vi "Describe Comparison.vi"(6 "Delta":variant, 9 "Actual":variant, 10 "Expected":variant) -> (2 "Description":string)   [LabVIEW 2020]
uses:
  <vilib>/Utility/Data Type/NI_Data Type.lvlib
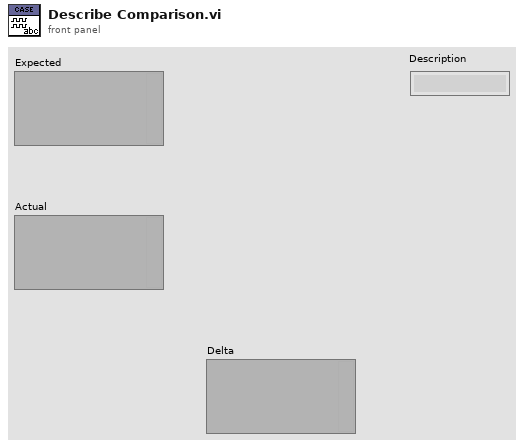
[diagram p1: front panel]
types:
  T1 = typedef "NI_Data Type.lvlib/Data Type.ctl" = enum8{"Invalid Type", "Void", "I8", "I16", "I32", "I64", "U8", "U16", "U32", "U64", "Single Float", "Double Float", "Extended Float", "Single Complex", "Double Complex", "Extended Complex", "Enum U8", "Enum U16", "Enum U32", "Enum U64", "Single Float With Unit", "Double Float With Unit", "Extended Float With Unit", "Single Complex with Unit", "Double Complex with Unit", "Extended Complex with Unit", "Boolean", "String", "Path", "Picture", "Tag", "Array", "Cluster", "Variant", "LV Variant", "Waveform", "Timestamp", "Digital Waveform", "Digital Data", "ExpressData", "Refnum", "External Data", "VI", "Poly VI", "LabVIEW Class Instance", "Fixed Point", "Set Collection", "Map Collection"}
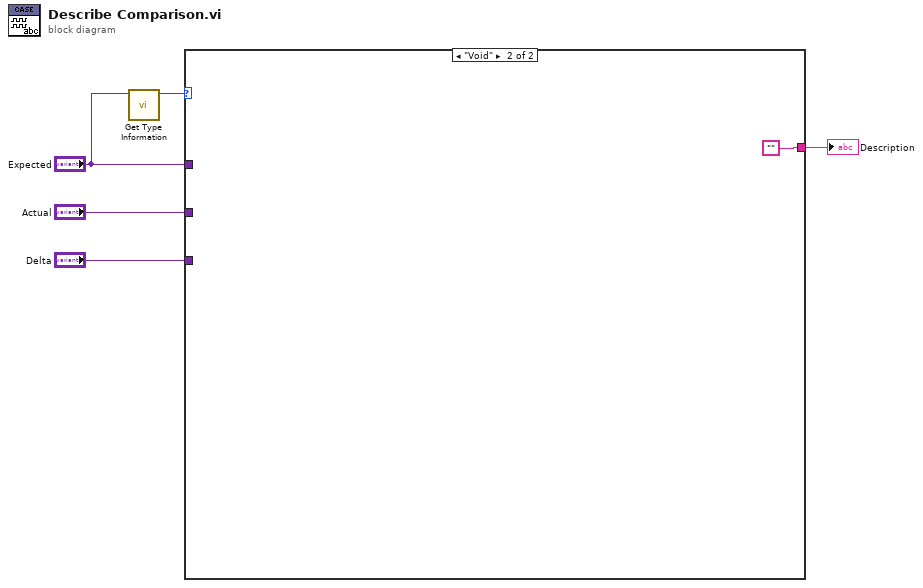
[diagram p0: block diagram]
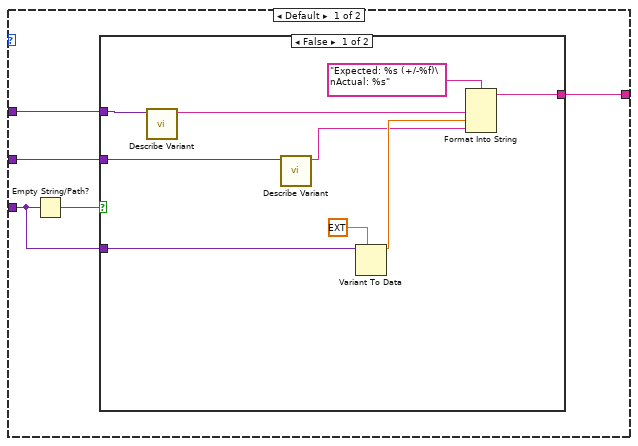
[diagram p2: hidden frame]
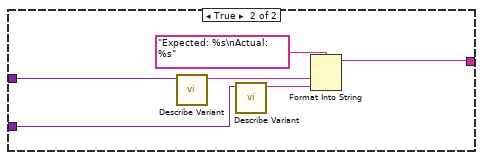
[diagram p3: hidden frame]
diagram:
  n1 = call <vilib>:"Get Type Information.vi"("variant"="Expected") -> ("type"=w1:T1)  [unwired: 6 in, 4 out]
  n2 = case shown="\"Void\"" w1 {
    tunnel: "Actual" -> [w10 _]
    tunnel: "Delta" -> [w8 _]
    tunnel: [w7 ""] -> w3
    tunnel: "Expected" -> [w6 _]
    frame Default {
      n3 = Empty String/Path?(string/path=w8) -> (empty?=w9:bool)
      n4 = case shown="False" w9 {
        tunnel: w6 -> [w16 w22]
        tunnel: w10 -> [w14 w21]
        tunnel: w8 -> [w15 _]
        tunnel: [w13 w20] -> w7
        frame False {
          n5 = call "Describe Variant.vi"("Variant"=w16) -> ("Variant Description"=w17:string)  [unwired: 8 in, 2 out]
          n6 = call "Describe Variant.vi"("Variant"=w14) -> ("Variant Description"=w11:string)  [unwired: 8 in, 2 out]
          n7 = Variant To Data(type=ext 0.0, Variant=w15) -> (data=w12:ext)  [unwired: 1 in, 1 out]
          n8 = Format Into String(format string="Expected: %s (+/-%f)\nActual: %s", w17, w12, w11) -> (resulting string=w13:string)  [unwired: 2 in, 1 out]
        }
        frame True {
          n9 = call "Describe Variant.vi"("Variant"=w22) -> ("Variant Description"=w25:string)  [unwired: 8 in, 2 out]
          n10 = call "Describe Variant.vi"("Variant"=w21) -> ("Variant Description"=w23:string)  [unwired: 8 in, 2 out]
          n11 = Format Into String(format string="Expected: %s\nActual:   %s", w25, w23) -> (resulting string=w20:string)  [unwired: 2 in, 1 out]
        }
      }
    }
    frame "Void" {
    }
  }
  "Description" <- w3
